vi "Create Temporary File.vi"(8 "error in (no error)":errorcluster) -> (0 "error out":errorcluster, 3 "Temp file path":path)   [LabVIEW 2016, in "Post Build Action Tester.lvclass"]
uses:
  Post Build Action Tester.lvclass
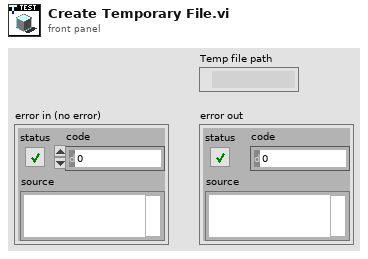
[diagram p1: front panel]
types:
  T1 = enum16{"open", "replace", "create", "open or create", "replace or create", "replace or create with confirmation"}
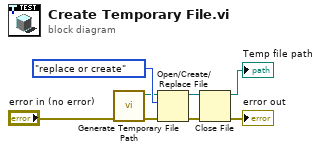
[diagram p0: block diagram]
diagram:
  n1 = call <vilib>:"Generate Temporary File Path.vi"("error in (no error)"="error in (no error)") -> ("error out"=w1:errorcluster, "Unique Temporary File Path"=w3:path)  [unwired: 9 in]
  n2 = Open/Create/Replace File(file path (use dialog)=w3, error in=w1, operation (0:open)=T1."replace or create") -> (refnum out=w6:refnum<file>, error out=w4:errorcluster)  [unwired: 3 in, 1 out]
  n3 = Close File(refnum=w6, error in=w4) -> (path=→"Temp file path":path, error out=→"error out":errorcluster)
